vi "Check increment toastedness.vi"(8 "Slow toast?":bool, 9 "Started last toasting stage":timestamp, 10 "Now":timestamp, 11 "Toast value":T1) -> (3 "Increment toastedness":bool)   [LabVIEW 2018, in "Toaster.lvlib"]
doc: "Checks whether the toast is ready to get browner, depending on whether it is toasting in normal mode or defrost/reheat."
uses:
  Toaster.lvlib
  controls/Toast.ctl
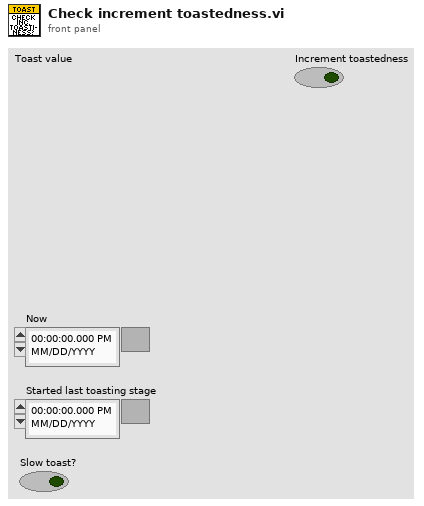
[diagram p1: front panel]
types:
  T1 = typedef "Toaster.lvlib/Toast.ctl" = enum32{"Empty", "Bread", "Toasting", "Toasted", "Burnt"}
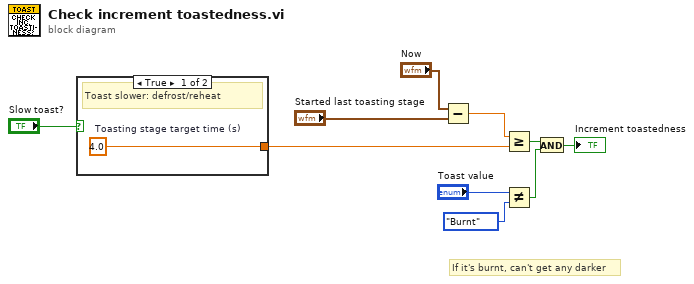
[diagram p0: block diagram]
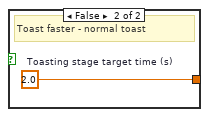
[diagram p2: hidden frame]
diagram:
  # "If it's burnt, can't get any darker"
  n1 = case shown="True" "Slow toast?" {
    tunnel: [w11 w12] -> w7
    frame True {
      w11 = 4.0  # Toasting stage target time (s)
      # "Toast slower: defrost/reheat"
    }
    frame False {
      w12 = 2.0  # Toasting stage target time (s)
      # "Toast faster - normal toast"
    }
  }
  n2 = Subtract(x="Now", y="Started last toasting stage") -> (x-y=w8:dbl)
  n3 = Greater Or Equal?(x=w8, y=w7) -> (x >= y?=w2:bool)
  n4 = Not Equal?(x="Toast value", y=Toast."Burnt" ("Value")) -> (x != y?=w4:bool)
  n5 = And(x=w2, y=w4) -> (x .and. y?=→"Increment toastedness":bool)
